vi "Write Value.vi"(8 "error in (no error)":errorcluster, 9 "Force draw? (F)":bool, 10 "New Value":T1, 11 "BetterTreeBar in":refnum<class "BetterHorizontalBar.lvclass">) -> (0 "error out":errorcluster, 3 "BetterTreeBar out":refnum<class "BetterHorizontalBar.lvclass">)   [LabVIEW 2020, in "BetterDragAndDrop.lvlib" / "BetterHorizontalBar.lvclass"]
uses:
  BetterHorizontalBar.lvclass
  SubVIs/Horizontal Bar Enumeration.ctl
  BetterHorizontalBar.lvclass/BetterHorizontalBar.ctl
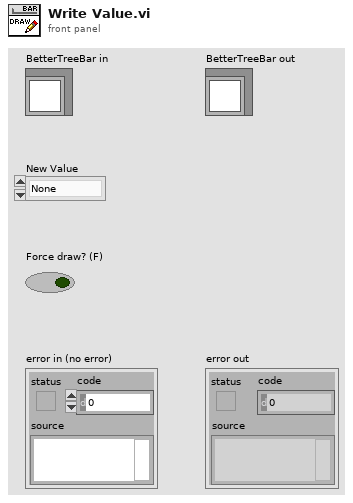
[diagram p1: front panel]
types:
  T1 = typedef "BetterDragAndDrop.lvlib/BetterHorizontalBar.lvclass/Horizontal Bar Enumeration.ctl" = enum16{"None", "only bar", "tilda up"}
  T2 = typedef "BetterDragAndDrop.lvlib/BetterTreeBar.lvclass/Horizontal Bar Enumeration.ctl" = enum16{"None", "only bar", "tilda up"}
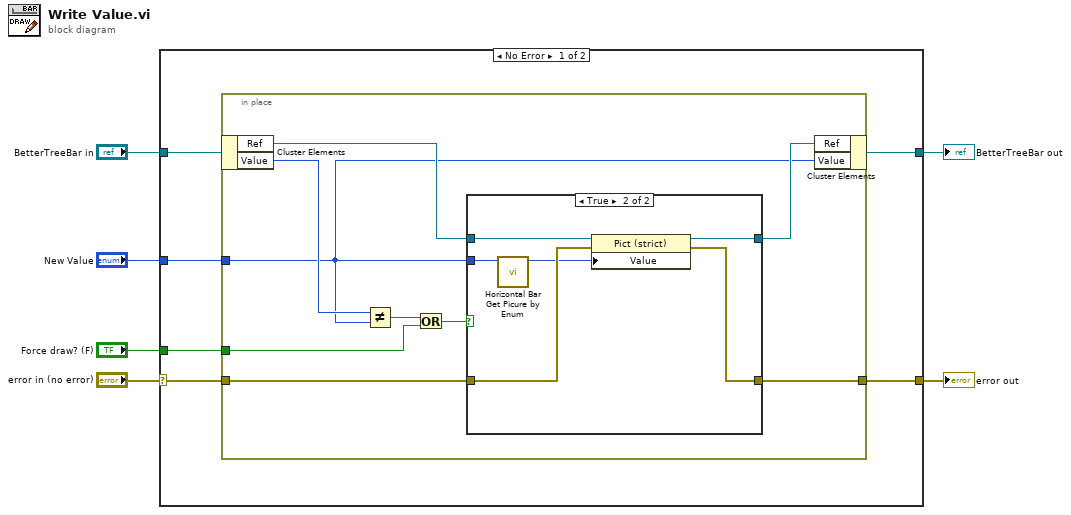
[diagram p0: block diagram]
diagram:
  n1 = case shown="No Error" "error in (no error)" {
    selector: "error in (no error)" -> [w8 w31]
    tunnel: [w7 w31] -> w5
    tunnel: [w11 w30] -> w3
    tunnel: "BetterTreeBar in" -> [w12 w30]
    tunnel: "New Value" -> [w10 _]
    tunnel: "Force draw? (F)" -> [w9 _]
    frame No Error {
      n2 = in-place {
        in-place-border: w10 -> [w13]
        in-place-border: w9 -> [w17]
        in-place-border: w8 -> [w15]
        in-place-border: [w14] -> w7
        n3 = in-place-cluster #1(w12) -> ("Ref"=w21:refnum<vi>, "Value"=w19:T2)
        n4 = Not Equal?(x=w19, y=w13) -> (x != y?=w18:bool)
        n5 = Or(x=w18, y=w17) -> (x .or. y?=w16:bool)
        n6 = case shown="True" w16 {
          tunnel: w21 -> [w23 w29]
          tunnel: [w23 w28] -> w20
          tunnel: w15 -> [w22 w27]
          tunnel: [w22 w26] -> w14
          tunnel: w13 -> [_ w25]
          frame False {
          }
          frame True {
            n7 = call "Horizontal Bar Get Picure by Enum.vi"("Type"=w25) -> ("value"=w24:picture)  [unwired: 10 in]
            n8 = property class="Pict (strict)"(reference=w29, error in=w27, "Value"=w24) -> (reference out=w28:refnum<vi>, error out=w26:errorcluster)
          }
        }
        n9 = in-place-cluster #1("Ref"=w20, "Value"=w13) -> (w11:refnum<class "BetterHorizontalBar.lvclass">)
      }
    }
    frame Error {
    }
  }
  "error out" <- w5
  "BetterTreeBar out" <- w3
